vi "37查看中壢市.vi"() -> ()   [LabVIEW 2014]
panel:
  in  "OK Button":bool
  in  "底色":u32(colorbox)=16768479
  # "中壢市"
  # "土地價格：1000"
  # "§Ú\n¬O\n¤¤\nÃc\n¤H\n¤£\n¬O\n®ç\n¶é\n¤H"
  # "蓋房子價格：500"
  # "蓋旅館價格：800"
  # "過路費"
  # "空地：300"
  # "一棟房子：+300"
  # "一棟旅館：+800"
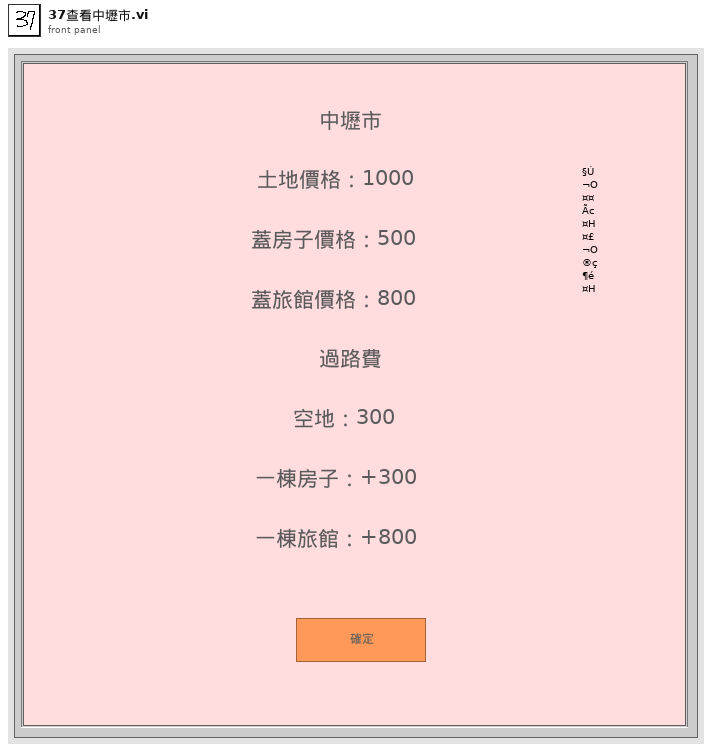
[diagram p1: front panel]
types:
  T1 = enum8{"Enabled", "Disabled", "Disabled and Grayed Out"}
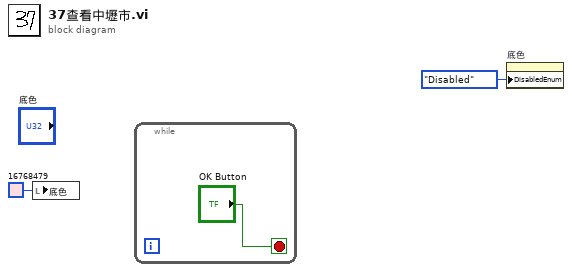
[diagram p0: block diagram]
diagram:
  n1 = local write "底色"(u32 16768479 ("底色")) -> ()
  n2 = while {
    stop <- "OK Button" stop-if-true
  }
  n3 = property on="底色" class="ColBox"("DisabledEnum"=T1."Disabled" ("Disabled")) -> ()  [unwired: 2 in, 2 out]
